vi "DAC Configure.vi"(8 "error in":errorcluster, 11 "DAC Keller Diff P 23X in":refnum<class "DAC Keller Diff P 23X.lvclass">) -> (0 "error out":errorcluster, 3 "DAC Keller Diff P 23X out":refnum<class "DAC Keller Diff P 23X.lvclass">)   [LabVIEW 2019, in "DAC.lvlib" / "DAC Keller Diff P 23X.lvclass"]
uses:
  DAC Keller Diff P 23X.lvclass
  C:/Users/krio/Documents/LV_Projects/test-stand/App/DAC/DAC.lvclass
  DAC.lvclass/DAC.ctl
  <instrlib>/_KELLER RS485 Library/Public/Type Definitions/Baud Rate.ctl
  DAC Keller Diff P 23X.lvclass/DAC Keller Diff P 23X.ctl
  <vilib>/Utility/error.llb/Error Cluster From Error Code.vi
  <vilib>/ErrorRing/Error Ring.xnode
  DAC.lvclass
  <instrlib>/_KELLER RS485 Library/KELLER RS485 Library.lvlib
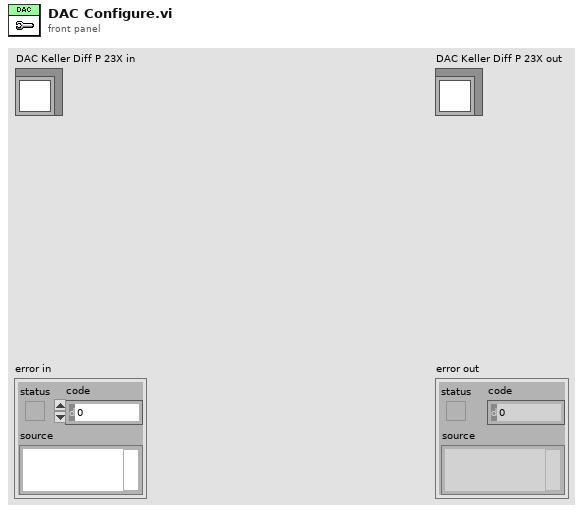
[diagram p1: front panel]
types:
  T1 = typedef "KELLER RS485 Library.lvlib/Baud Rate.ctl" = enum16{"9600bd", "115200bd"}
  T2 = typedef "KELLER RS485 Library.lvlib/Bus.ctl" = cluster{"VISA":refnum<visa-resource-name>, "Baud Rate ":T1, "Timeout":u32, "Echo?":bool, "Wait before transmit":u32}
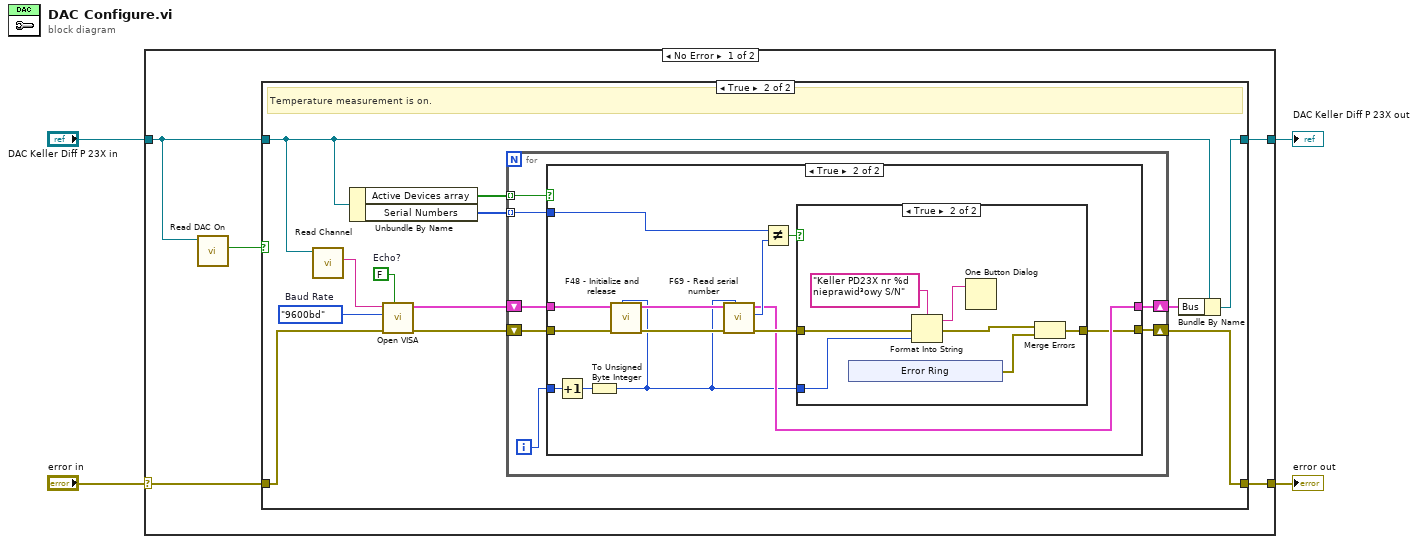
[diagram p0: block diagram]
diagram:
  n1 = case shown="No Error" "error in" {
    selector: "error in" -> [w6 w60]
    tunnel: [w5 w60] -> w4
    tunnel: [w7 w59] -> w3
    tunnel: "DAC Keller Diff P 23X in" -> [w9 w59]
    frame No Error {
      n2 = call "Read DAC On.vi"("DAC in"=w9) -> ("DAC On"=w8:bool)  [unwired: 8 in, 2 out]
      n3 = case shown="True" w8 {
        tunnel: w9 -> [w11 w20]
        tunnel: [w11 w23] -> w7
        tunnel: w6 -> [w10 w19]
        tunnel: [w10 w17] -> w5
        frame False {
          # "Temperature measurement is off."
        }
        frame True {
          w12 = FALSE  # Echo?
          w21 = Baud_Rate."9600bd"  # Baud Rate
          # "Temperature measurement is on."
          n4 = call "Read Channel.vi"("DAC in"=w20) -> ("Channel"=w22:string)  [unwired: 8 in, 2 out]
          n5 = Unbundle By Name(w20) -> ("Active Devices array"=w14:bool[], "Serial Numbers"=w13:u32[])
          n6 = call <instrlib>:"Open VISA.vi"("Echo? (T)"=w12, "error in (no error)"=w19, "Baud Rate (9600bd)"=w21, "VISA resource name"=w22) -> ("error out"=w15:errorcluster, "Bus out"=w16:T2)  [unwired: 6 in]
          n7 = for {
            tunnel: w14 -> [w30] mode=indexing
            tunnel: w13 -> [w26] mode=indexing
            shift-right: [w24] -> w17
            shift-left: w15 -> [w27]
            shift-right: [w25] -> w18
            shift-left: w16 -> [w28]
            i -> [w29]
            n8 = case shown="True" w30 {
              tunnel: w29 -> [_ w45]
              tunnel: w28 -> [w32 w37]
              tunnel: w27 -> [w31 w36]
              tunnel: w26 -> [_ w42]
              tunnel: [w32 w39] -> w25
              tunnel: [w31 w38] -> w24
              frame False {
              }
              frame True {
                n9 = Increment(x=w45) -> (x+1=w44:i32)
                n10 = To Unsigned Byte Integer(number=w44) -> (unsigned 8bit integer=w33:u8)
                n11 = call <instrlib>:"F48 - Initialize and release.vi"("Address (250)"=w33, "error in (no error)"=w36, "Bus in"=w37) -> ("error out"=w34:errorcluster, "Bus out"=w35:T2)  [unwired: 5 in, 2 out]
                n12 = call <instrlib>:"F69 - Read serial number.vi"("Address (250)"=w33, "error in (no error)"=w34, "Bus in"=w35) -> ("error out"=w40:errorcluster, "Serial number out"=w43:u32, "Bus out"=w39:T2)  [unwired: 6 in]
                n13 = Not Equal?(x=w42, y=w43) -> (x != y?=w41:bool)
                n14 = case shown="True" w41 {
                  tunnel: w33 -> [_ w52]
                  tunnel: w40 -> [w46 w50]
                  tunnel: [w46 w47] -> w38
                  frame False {
                  }
                  frame True {
                    n15 = xnode "Error Ring"() -> ("error out"=w48:errorcluster)
                    n16 = Format Into String(format string="Keller PD23X nr %d nieprawid³owy S/N", error in=w50, w52) -> (resulting string=w51:string, error out=w49:errorcluster)  [unwired: 1 in]
                    n17 = One Button Dialog(message=w51) -> ()  [unwired: 1 in, 1 out]
                    n18 = Merge Errors(w49, w48) -> (w47:errorcluster)
                  }
                }
              }
            }
          }
          n19 = Bundle By Name(cluster=w20, "Bus"=w18) -> (w23:refnum<class "DAC Keller Diff P 23X.lvclass">)
        }
      }
    }
    frame Error {
    }
  }
  "error out" <- w4
  "DAC Keller Diff P 23X out" <- w3
